vi "uA_change_shunt_res_without_lose_power.vi"(8 "error in":errorcluster, 10 "Shunt Slector":enum16{"Shunt 3.333 Ohm", "Shunt 1 Ohm"}(ring), 11 "device name":tag) -> (0 "error out":errorcluster)   [LabVIEW 2015]
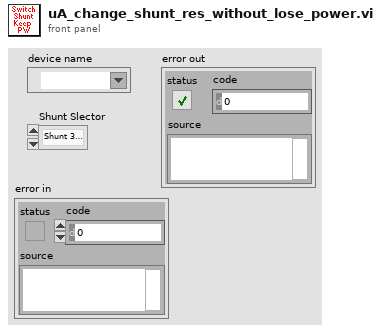
[diagram p1: front panel]
types:
  T1 = enum16{"Turn On bypass - Off Shunt", "Turn Off bypass - On Shunt"}
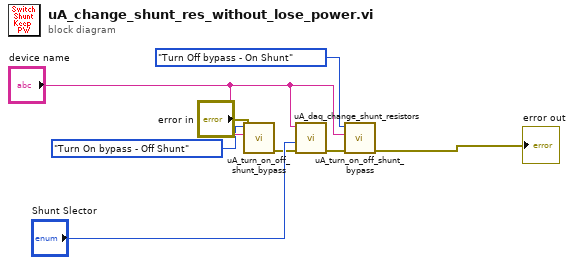
[diagram p0: block diagram]
diagram:
  n1 = call "uA_turn_on_off_shunt_bypass.vi"("error in"="error in", "USB DAQ"="device name", "Bypass Shunt"=T1."Turn On bypass - Off Shunt") -> ("error out"=w3:errorcluster)  [unwired: 8 in]
  n2 = call "uA_daq_change_shunt_resistors.vi"("error in"=w3, "Shunt Slector"="Shunt Slector", "device name"="device name") -> ("error out"=w2:errorcluster)  [unwired: 8 in]
  n3 = call "uA_turn_on_off_shunt_bypass.vi"("error in"=w2, "USB DAQ"="device name", "Bypass Shunt"=T1."Turn Off bypass - On Shunt") -> ("error out"=→"error out":errorcluster)  [unwired: 8 in]
